vi "Get current position.vi"(8 "error in (no error)":errorcluster, 11 "Position arguments":T1) -> (0 "error out":errorcluster, 1 "Keep moving?":bool, 2 "Acquiring?":bool, 3 "Position out":cluster{"M1 pos":dbl, "M2 pos ":dbl})   [LabVIEW 2020]
doc: "Calculates the current position of the motors and returns whether acquisition should continue or stop."
uses:
  NI_DAQ/Libraries/NI DAQ/NI DAQ.lvlib
  controls/Motor direction ---typedef.ctl
  controls/Position arguments ---typedef.ctl
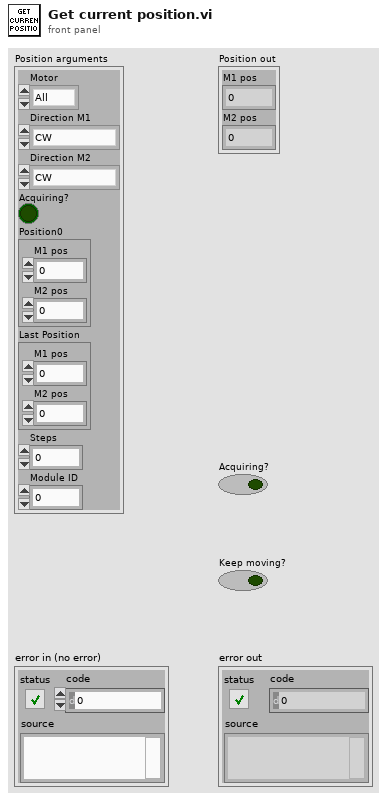
[diagram p1: front panel]
types:
  T1 = typedef "Position arguments ---typedef.ctl" = cluster{"Motor":enum16{"All", "M1", "M2"}, "Direction M1":T2, "Direction M2":T2, "Acquiring?":bool, "Position0":cluster{"M1 pos":dbl, "M2 pos ":dbl}, "Last Position":cluster{"M1 pos":dbl, "M2 pos ":dbl}, "Steps":i32, "Module ID":i32}
  T2 = typedef "Motor direction ---typedef.ctl" = enum16{"CW", "CCW", "IDLE"}
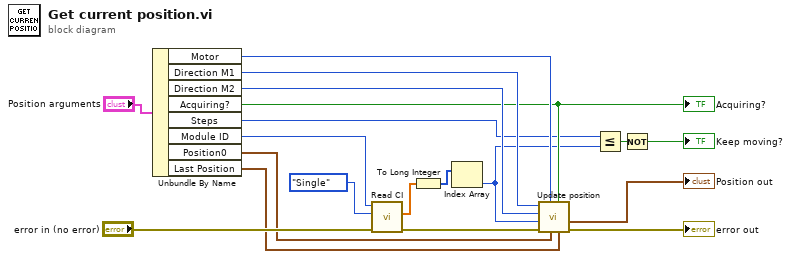
[diagram p0: block diagram]
diagram:
  n1 = Unbundle By Name("Position arguments") -> ("Motor"=w10:enum16{"All", "M1", "M2"}, "Direction M1"=w9:T2, "Direction M2"=w8:T2, "Acquiring?"=w7:bool, "Steps"=w6:i32, "Module ID"=w5:i32, "Position0"=w2:cluster{"M1 pos":dbl, "M2 pos ":dbl}, "Last Position"=w1:cluster{"M1 pos":dbl, "M2 pos ":dbl})
  "Acquiring?" <- w7
  n2 = call "Read CI.vi"("error in"="error in (no error)", "Samples"=enum16{"Single", "Multiple"}."Single", "Module ID"=w5) -> ("error out"=w13:errorcluster, "data"=w14:dbl[])  [unwired: 6 in, 1 out]
  n3 = To Long Integer(number=w14) -> (32bit integer=w15:i32[])
  n4 = Index Array(array=w15) -> (element=w3:i32)  [unwired: 1 in]
  n5 = call "Update position.vi"("Last position"=w1, "Acquiring?"=w7, "Position 0"=w2, "Motor"=w10, "error in (no error)"=w13, "Steps taken"=w3, "Direction M2"=w8, "Direction M1"=w9) -> ("error out"=→"error out":errorcluster, "Position out"=→"Position out":cluster{"M1 pos":dbl, "M2 pos ":dbl})  [unwired: 2 in]
  n6 = Less Or Equal?(x=w6, y=w3) -> (x <= y?=w17:bool)
  n7 = Not(x=w17) -> (.not. x?=→"Keep moving?":bool)
